vi "Create Session Connect Event.vi"(8 "error in (no error)":errorcluster, 11 "gRPC Server in":refnum<class "gRPC Server.lvclass">) -> (0 "error out":errorcluster, 1 "Session Connect gRPC UE":refnum<user-event>, 2 "New Session":refnum<user-event>, 3 "gRPC Server out":refnum<class "gRPC Server.lvclass">)   [LabVIEW 2019, in "gRPC Server (template.proto).lvlib" / "gRPC Server.lvclass"]
uses:
  gRPC Server.lvclass
  <vilib>/gRPC/LabVIEW gRPC Library/Shared/grpcId.ctl
  <vilib>/gRPC/LabVIEW gRPC Library/grpc-lvsupport-release.lvlib
  <vilib>/gRPC/LabVIEW gRPC Library/Server API/typeDefs/gRPCId Cluster.ctl
  <vilib>/gRPC/LabVIEW gRPC Servicer/ServiceBase/ServiceBase.lvclass
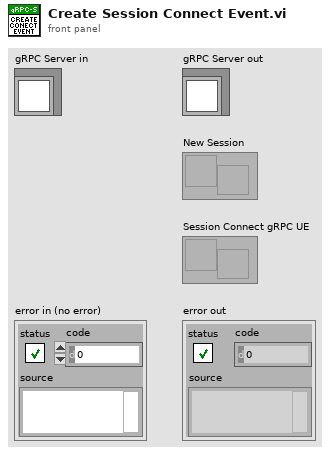
[diagram p1: front panel]
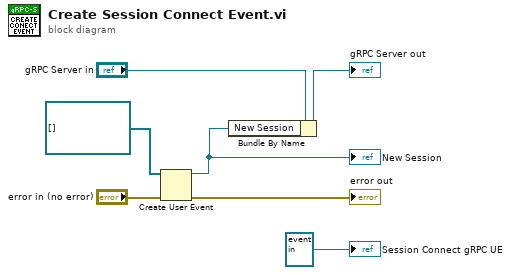
[diagram p0: block diagram]
diagram:
  n1 = Create User Event(user event datatype=refnum<class "ServiceBase.lvclass">[] [] ("gRPC services out"), error in="error in (no error)") -> (user event=w2:refnum<user-event>, error out=→"error out":errorcluster)
  "New Session" <- w2
  n2 = Bundle By Name(cluster="gRPC Server in", "New Session"=w2) -> (→"gRPC Server out":refnum<class "gRPC Server.lvclass">)
  "Session Connect gRPC UE" <- refnum<user-event> refnum ("Session Connect gRPC UE")
